vi "SRV_Get Sensor View ref From Selection.vi"(5 "Sensor View refs":T1, 9 "Sensor View":T2, 11 "error in (no error)":errorcluster) -> (2 "Boolean ref?":bool, 3 "Knob ref?":bool, 8 "Selected ref":refnum<vi>, 10 "Valid ref?":bool, 15 "error out":errorcluster)   [LabVIEW 2014]
uses:
  SRV_Sensors Names.ctl
  SRV_Sensor View refs.ctl
panel:
  out "Index within Array":i32
  out "Array Index":i32
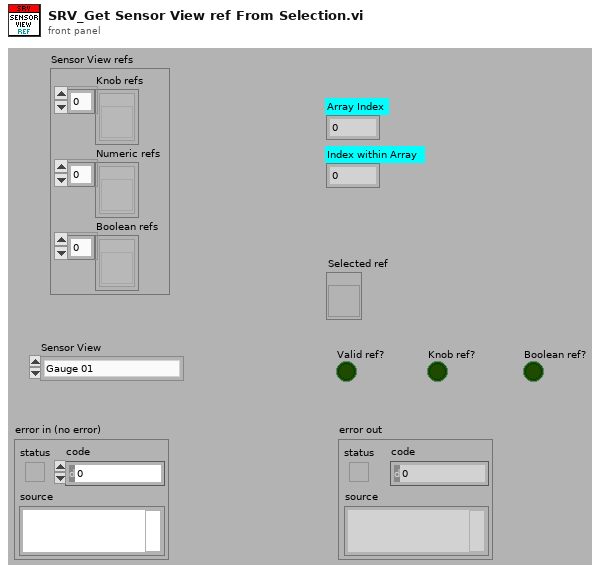
[diagram p1: front panel]
types:
  T1 = typedef "SRV_Sensor View refs.ctl" = cluster{"Knob refs":refnum<vi>[], "Numeric refs":refnum<vi>[], "Boolean refs":refnum<vi>[]}
  T2 = typedef "SRV_Sensors Names.ctl" = enum16{"Gauge 01", "Gauge 02", "Gauge 03", "Gauge 04", "Meter 01", "Meter 02", "Meter 03", "Meter 04", "Numeric 01", "Numeric 02", "Numeric 03", "Numeric 04", "Numeric 05", "Numeric 06", "Numeric 07", "Numeric 08", "Boolean 01", "Boolean 02", "Boolean 03", "Boolean 04", "Boolean 05", "Boolean 06", "Boolean 07", "Boolean 08", "Boolean 09", "Boolean 10", "Boolean 11", "Boolean 12", "Boolean 13", "Boolean 14", "Boolean 15", "Boolean 16", "Boolean 17", "Boolean 18", "Boolean 19", "Boolean 20", "Boolean 21", "Boolean 22", "Boolean 23", "Boolean 24", "Boolean 25", "Boolean 26", "Boolean 27", "Boolean 28", "Boolean 29", "Boolean 30", "Boolean 31", "Boolean 32"}
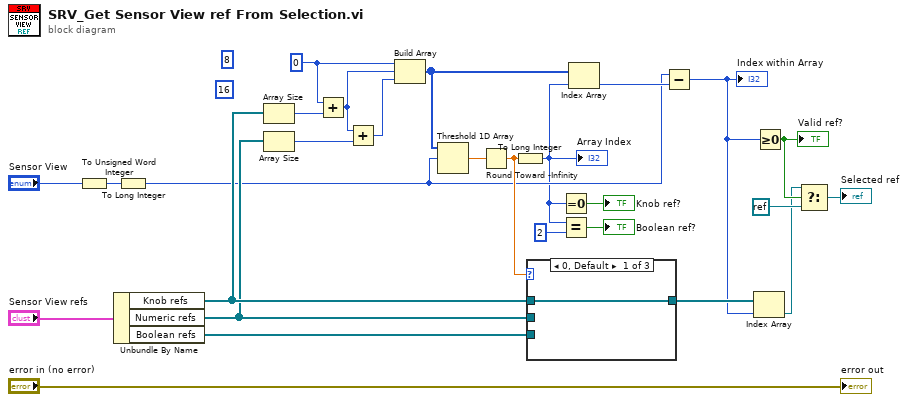
[diagram p0: block diagram]
diagram:
  (unwired) 16 ("size(s)")
  (unwired) 8 ("size(s)")
  w10 = 0 ("size(s)")
  n1 = To Unsigned Word Integer(number="Sensor View") -> (unsigned 16bit integer=w26:u16)
  n2 = Unbundle By Name("Sensor View refs") -> ("Knob refs"=w23:refnum<vi>[], "Numeric refs"=w21:refnum<vi>[], "Boolean refs"=w20:refnum<vi>[])
  n3 = To Long Integer(number=w26) -> (32bit integer=w4:i32)
  n4 = Array Size(array=w23) -> (size(s)=w9:i32)
  n5 = Array Size(array=w21) -> (size(s)=w7:i32)
  n6 = Add(x=w10, y=w9) -> (x+y=w8:i32)
  n7 = Add(x=w8, y=w7) -> (x+y=w6:i32)
  n8 = Build Array(w10, w8, w6) -> (w19:i32[])
  n9 = Threshold 1D Array(2:w4, 3:w19) -> (0:w24:dbl)  [unwired: 1 in]
  n10 = Round Toward -Infinity(1:w24) -> (0:w22:dbl)
  n11 = To Long Integer(number=w22) -> (32bit integer=w2:i32)
  "Array Index" <- w2
  n12 = case shown="0, Default" w22 {
    tunnel: w23 -> [w28 _ _]
    tunnel: w21 -> [_ w29 _]
    tunnel: w20 -> [_ _ w30]
    tunnel: [w28 w29 w30] -> w17
    frame 0, Default {
    }
    frame 1 {
    }
    frame 2 {
    }
  }
  n13 = Equal To 0?(x=w2) -> (x = 0?=→"Knob ref?":bool)
  n14 = Equal?(x=w2, y=2) -> (x = y?=→"Boolean ref?":bool)
  n15 = Index Array(array=w19, index=w2) -> (element=w18:i32)
  n16 = Subtract(x=w4, y=w18) -> (x-y=w14:i32)
  "Index within Array" <- w14
  n17 = Index Array(array=w17, index=w14) -> (element=w11:refnum<vi>)
  n18 = Greater Or Equal To 0?(x=w14) -> (x >= 0?=w13:bool)
  "Valid ref?" <- w13
  n19 = Select(t=w11, s=w13, f=refnum<k0> refnum) -> (s? t:f=→"Selected ref":refnum<vi>)
  "error out" <- "error in (no error)"
